vi "toTimestamp.vi"(9 "Fractional Second":dbl format="%#.6f", 10 "System Time (s)":i64, 11 "Epoch (Local)":refnum<class "Epoch.lvclass">) -> (1 "Not a Timestamp?":bool, 2 "Timestamp":timestamp, 3 "Epoch (out)":refnum<class "Epoch.lvclass">)   [LabVIEW 2013, in "Epoch.lvclass"]
uses:
  Epoch.lvclass
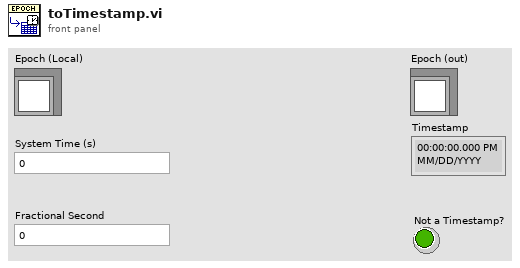
[diagram p1: front panel]
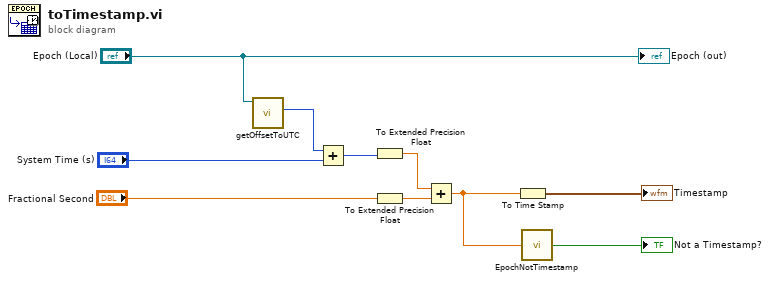
[diagram p0: block diagram]
diagram:
  n1 = call-dynamic "getOffsetToUTC.vi"("Epoch"="Epoch (Local)") -> ("Offset to UTC"=w5:i64)  [unwired: 10 in]
  n2 = Add(x=w5, y="System Time (s)") -> (x+y=w4:i64)
  n3 = To Extended Precision Float(1:w4) -> (0:w8:ext)
  n4 = To Extended Precision Float(1:"Fractional Second") -> (0:w9:ext)
  n5 = Add(x=w8, y=w9) -> (x+y=w3:ext)
  n6 = To Time Stamp(1:w3) -> (0:→"Timestamp":timestamp)
  n7 = call "EpochNotTimestamp.vi"("Epoch Time"=w3) -> ("Not a Timestamp?"=→"Not a Timestamp?":bool)  [unwired: 8 in]
  "Epoch (out)" <- "Epoch (Local)"
